vi "Configure Programmer Setup Parameters.vi"(0 "VISA resource name":refnum<visa-resource-name>, 1 "Unit Address (1)":u8=1, 5 "PV Input (0)":i16, 7 "Setpoint Input (0)":i16, 9 "Enable Advance Segment (False)":bool, 11 "error in (no error)":errorcluster, 12 "Enable Skip Segment (False)":bool, 13 "Enable Synchronize Input (False)":bool) -> (4 "VISA resource name out":refnum<visa-resource-name>, 15 "error out":errorcluster)   [LabVIEW 2014, in "Eurotherm 35xx Series.lvlib"]
doc: "This VI configure Programmer Setup Parameters."
uses:
  <instrlib>/Eurotherm 35xx Series/Eurotherm 35xx Series.lvlib
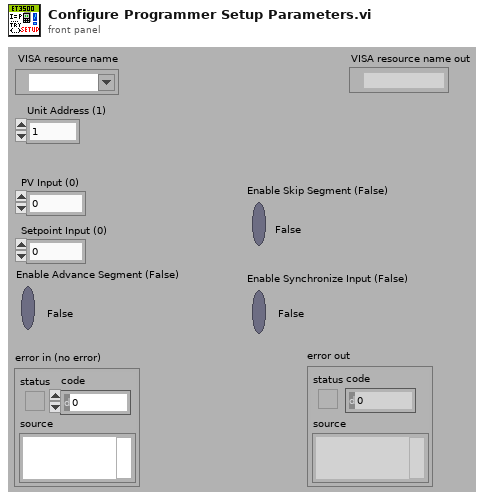
[diagram p1: front panel]
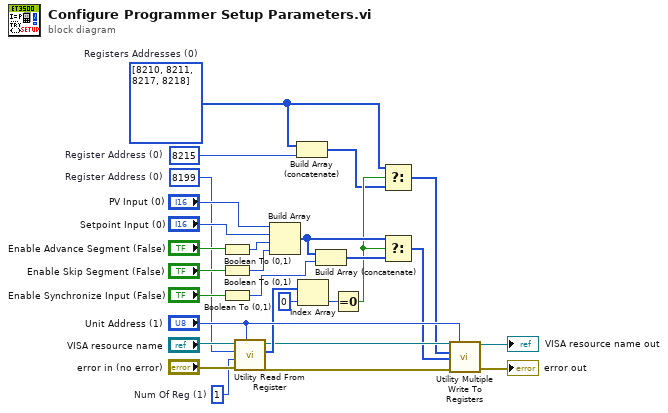
[diagram p0: block diagram]
diagram:
  w3 = 8215  # Register Address (0)
  w4 = 8199  # Register Address (0)
  w23 = u16 1  # Num Of Reg (1)
  w5 = u16[] [8210, 8211, 8217, 8218]  # Registers Addresses (0)
  n1 = Boolean To (0,1)(Boolean="Enable Advance Segment (False)") -> (0, 1=w13:i16)
  n2 = Boolean To (0,1)(Boolean="Enable Skip Segment (False)") -> (0, 1=w12:i16)
  n3 = Boolean To (0,1)(Boolean="Enable Synchronize Input (False)") -> (0, 1=w8:i16)
  n4 = call <instrlib>:"Utility Read From Register.vi"("Unit Address (1)"="Unit Address (1)", "error in (no error)"="error in (no error)", "Num Of Reg (1)"=w23, "Register Address (0)"=w4, "VISA resource name"="VISA resource name") -> ("error out"=w20:errorcluster, "Data"=w22:i16[], "VISA resource name out"=w21:refnum<visa-resource-name>)  [unwired: 4 in]
  n5 = Build Array("PV Input (0)", "Setpoint Input (0)", w13, w12) -> (w10:i16[])
  n6 = Build Array (concatenate)(w5, w3) -> (w6:i32[])
  n7 = Index Array(array=w22, index=0) -> (element=w11:i16)
  n8 = Build Array (concatenate)(w10, w8) -> (w9:i16[])
  n9 = Equal To 0?(x=w11) -> (x = 0?=w7:bool)
  n10 = Select(t=w5, s=w7, f=w6) -> (s? t:f=w2:i32[])
  n11 = Select(t=w10, s=w7, f=w9) -> (s? t:f=w1:i16[])
  n12 = call <instrlib>:"Utility Multiple Write To Registers.vi"("VISA resource name"=w21, "Unit Address (1)"="Unit Address (1)", "Registers Addresses (0)"=w2, "Data (0)"=w1, "error in (no error)"=w20) -> ("VISA resource name out"=→"VISA resource name out":refnum<visa-resource-name>, "error out"=→"error out":errorcluster)  [unwired: 9 in]
